vi "Rumble Joystick 0 or Joystick 1.vi"(8 "error in (no error)":errorcluster, 9 "Joystick 0?":bool, 10 "Magnitude of buzz":sgl) -> (0 "error out":errorcluster)   [LabVIEW 2017]
uses:
  <vilib>/Rock Robotics/WPI/Utilities/WPI_GetSetVariantRefNum.vi
panel:
  # "rumble controler on Joysick"
  # "true: joystick 0\nfalse: joystick 1"
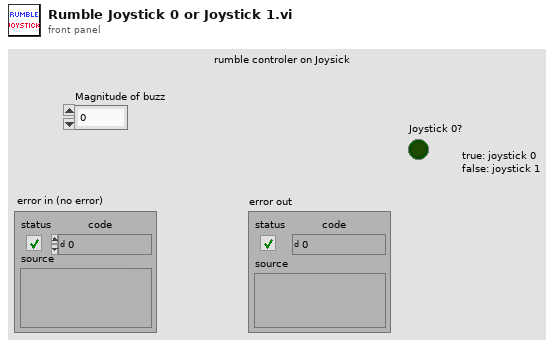
[diagram p1: front panel]
types:
  T1 = typedef "WPI_JoystickDevRef.ctl" = cluster{"Device":T2}
  T2 = typedef "WPI_JoystickDeviceEnum.ctl" = enum16{"USB 0", "USB 1", "USB 2", "USB 3", "USB 4", "USB 5"}
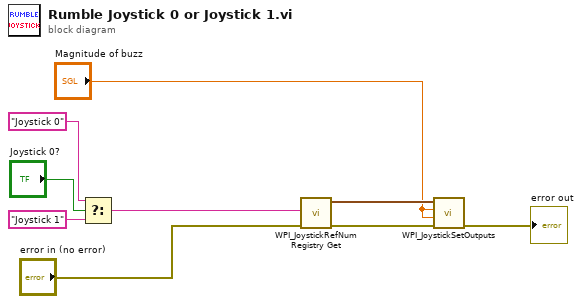
[diagram p0: block diagram]
diagram:
  n1 = Select(t="Joystick 0", s="Joystick 0?", f="Joystick 1") -> (s? t:f=w2:string)
  n2 = call <vilib>:"WPI_JoystickRefNum Registry Get.vi"("error in (no error)"="error in (no error)", "refnum name"=w2) -> ("error out"=w7:errorcluster, "JoystickDevRef"=w9:T1)  [unwired: 8 in]
  n3 = call <vilib>:"WPI_JoystickSetOutputs.vi"("error in (no error)"=w7, "Right Rumble"="Magnitude of buzz", "Left Rumble"="Magnitude of buzz", "JoystickDevRef"=w9) -> ("error out"=→"error out":errorcluster)  [unwired: 6 in, 1 out]
